vi "Insight_Measure_DataStreaming_FFT_Enable.vi"(8 "error in (no error)":errorcluster, 9 "Mode (Read / Write)":enum8{"Write", "Read"}(ring), 10 "Streaming FFT (On)":enum16{"Off", "On"}(ring)=enum."On", 11 "telnet connection":T1) -> (0 "error out":errorcluster, 1 "Streaming FFT?":enum16{"Off", "On"}(ring), 2 "response data":string, 3 "telnet  connection out":T1)   [LabVIEW 2011]
doc: "Insight Photonic Solutions\n\nThis VI enables or disables Data Streaming when the laser is in Measurement Mode.\n\nver 1.0 - original release\nver 3.3 - modifed to work with Atlas ver 3.3"
uses:
  Telnet Session.ctl
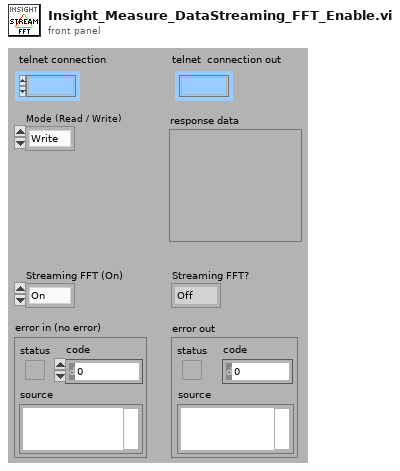
[diagram p1: front panel]
types:
  T1 = typedef "Telnet Session.ctl" = refnum<k1>
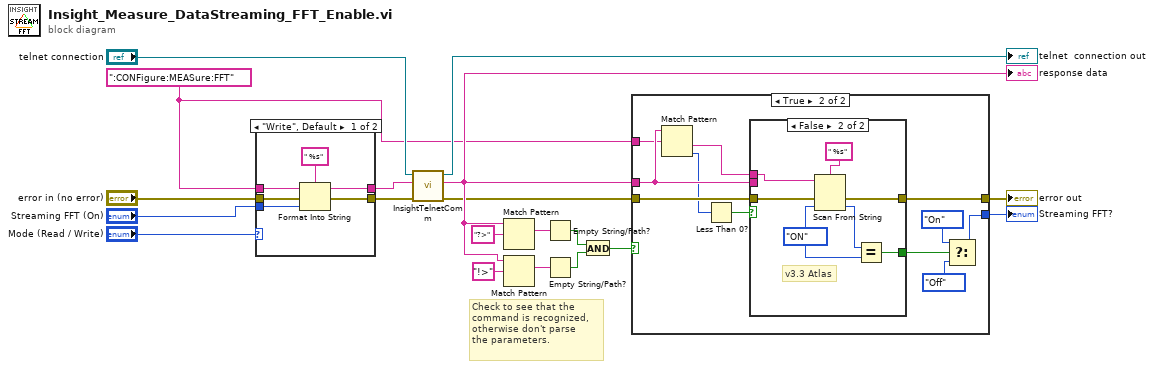
[diagram p0: block diagram]
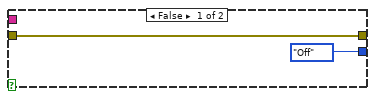
[diagram p2: hidden frame]
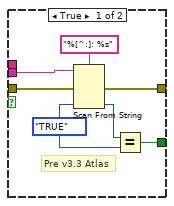
[diagram p3: hidden frame]
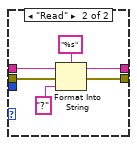
[diagram p4: hidden frame]
diagram:
  w1 = ":CONFigure:MEASure:FFT" ("String")
  # "Check to see that the \ncommand is recognized,\notherwise don't parse \nthe parameters."
  n1 = case shown="\"Write\", Default" "Mode (Read / Write)" {
    tunnel: [w25 w27] -> w17
    tunnel: "error in (no error)" -> [w24 w26]
    tunnel: w1 -> [w23 w29]
    tunnel: "Streaming FFT (On)" -> [w22 _]
    tunnel: [w20 w28] -> w16
    frame "Write", Default {
      n2 = Format Into String(format string=" %s", initial string=w23, error in=w24, w22) -> (resulting string=w20:string, error out=w25:errorcluster)
    }
    frame "Read" {
      n3 = Format Into String(format string="%s", initial string=w29, error in=w26, "?" ("input 1")) -> (resulting string=w28:string, error out=w27:errorcluster)
    }
  }
  n4 = call "InsightTelnetComm.vi"("error in"=w17, "write buffer (\"\")"=w16, "telnet connection"="telnet connection") -> ("error out"=w5:errorcluster, "response data"=w6:string, "telnet  connection out"=→"telnet  connection out":T1)  [unwired: 4 in]
  "response data" <- w6
  n5 = Match Pattern(string=w6, regular expression="?>") -> (match substring=w11:string)  [unwired: 1 in, 3 out]
  n6 = Match Pattern(string=w6, regular expression="!>") -> (match substring=w10:string)  [unwired: 1 in, 3 out]
  n7 = Empty String/Path?(string/path=w11) -> (empty?=w8:bool)
  n8 = Empty String/Path?(string/path=w10) -> (empty?=w7:bool)
  n9 = And(x=w8, y=w7) -> (x .and. y?=w2:bool)
  n10 = case shown="True" w2 {
    tunnel: [w33 w44] -> w4
    tunnel: w5 -> [w33 w43]
    tunnel: [enum16{"Off", "On"}."Off" ("Data Streaming (Off)") w41] -> w3
    tunnel: w6 -> [_ w38]
    tunnel: w1 -> [_ w37]
    frame False {
    }
    frame True {
      n11 = Match Pattern(string=w38, regular expression=w37) -> (after substring=w34:string, offset past match=w35:i32)  [unwired: 1 in, 2 out]
      n12 = Less Than 0?(x=w35) -> (x < 0?=w36:bool)
      n13 = case shown="False" w36 {
        tunnel: [w50 w57] -> w44
        tunnel: w43 -> [w49 w56]
        tunnel: w38 -> [w48 _]
        tunnel: [w47 w55] -> w42
        tunnel: w34 -> [_ w54]
        frame True {
          w45 = enum16{"FALSE", "TRUE"}."TRUE" ("Data Streaming")
          # "Pre v3.3 Atlas"
          n14 = Scan From String(format string="%[^:]: %s", input string=w48, error in=w49, default 2=w45) -> (error out=w50:errorcluster, output 2=w46:enum16{"FALSE", "TRUE"})  [unwired: 3 in, 2 out]
          n15 = Equal?(x=w46, y=w45) -> (x = y?=w47:bool)
        }
        frame False {
          w53 = enum16{"OFF", "ON"}."ON" ("Data Streaming")
          # "v3.3 Atlas"
          n16 = Scan From String(format string=" %s", input string=w54, error in=w56, default 1=w53) -> (error out=w57:errorcluster, output 1=w52:enum16{"OFF", "ON"})  [unwired: 1 in, 2 out]
          n17 = Equal?(x=w52, y=w53) -> (x = y?=w55:bool)
        }
      }
      n18 = Select(t=enum16{"Off", "On"}."On" ("Data Streaming (Off)"), s=w42, f=enum16{"Off", "On"}."Off" ("Data Streaming (Off)")) -> (s? t:f=w41:enum16{"Off", "On"})
    }
  }
  "error out" <- w4
  "Streaming FFT?" <- w3
